vi "read_channels_specify_range.vi"(5 "postDAQ  wait ms":u32=12, 7 "preDAQ  wait ms":u32=25, 8 "error in":T1, 11 "K6517 GPIB Address":string) -> (0 "error out":T1, 2 "data":dbl[](array[numeric]), 3 "K6517 GPIB Address out":string)   [LabVIEW 2024]
uses:
  <instrlib>/Keithley 6517/Keithley 6517.lvlib
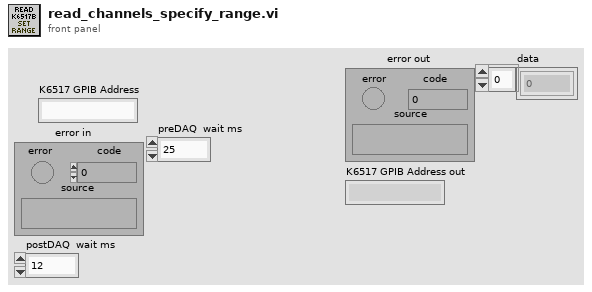
[diagram p1: front panel]
types:
  T1 = cluster{"error":bool, "code":i32, "source":string}
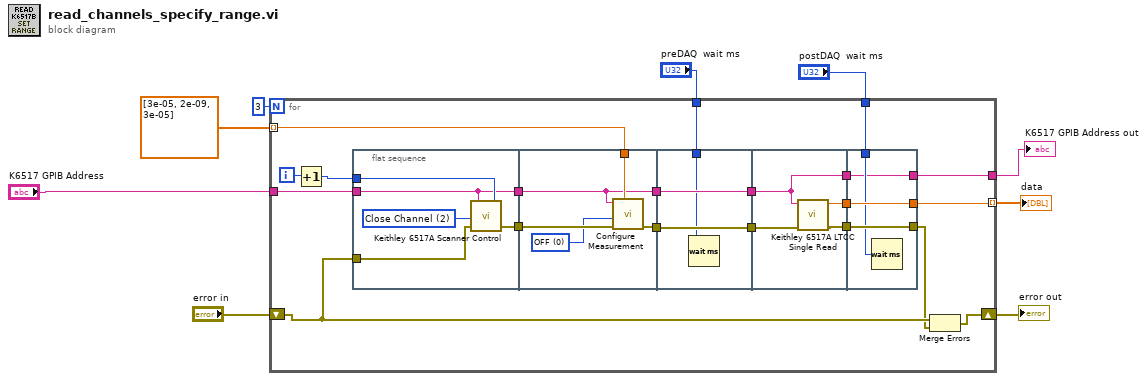
[diagram p0: block diagram]
diagram:
  n1 = for {
    N: 3 -> [_]
    tunnel: "K6517 GPIB Address" -> [w26]
    shift-right: [w29] -> w2
    shift-left: "error in" -> [w25]
    tunnel: dbl[] [3e-05, 2e-09, 3e-05] -> [w24] mode=indexing
    tunnel: [w14] -> w3 mode=indexing
    tunnel: "preDAQ  wait ms" -> [w13]
    tunnel: "postDAQ  wait ms" -> [w12]
    tunnel: [w11] -> w1
    i -> [w28]
    n2 = Increment(x=w28) -> (x+1=w27:i32)
    n3 = flat-sequence {
      tunnel: w27 -> [w33]
      tunnel: w26 -> [w31]
      tunnel: w25 -> [w32]
      tunnel: [w31] -> w23
      tunnel: [w30] -> w22
      tunnel: w24 -> [w37]
      tunnel: [w36] -> w20
      tunnel: [w35] -> w18
      tunnel: w22 -> [w39]
      tunnel: w23 -> [w35]
      tunnel: w20 -> [w42]
      tunnel: [w42] -> w19
      tunnel: w18 -> [w41]
      tunnel: [w41] -> w17
      tunnel: w13 -> [w40]
      tunnel: w19 -> [w46]
      tunnel: w17 -> [w43]
      tunnel: [w45] -> w21
      tunnel: [w44] -> w15
      tunnel: [w43] -> w10
      tunnel: [w50] -> w16
      tunnel: w21 -> [w50]
      tunnel: [w49] -> w14
      tunnel: w15 -> [w49]
      tunnel: w12 -> [w48]
      tunnel: [w47] -> w11
      tunnel: w10 -> [w47]
      frame #0 {
        w34 = u16 2 items=["Open All", "Open Channel", "Close Channel", "Scan List"] ("Scanner Control")
        n4 = call "Keithley 6517A Scanner Control.vi"("Open / Close Internal Scanner Channel"=w33, "error in"=w32, "Scanner Control"=w34, "GPIB address"=w31) -> ("error out"=w30:T1)  [unwired: 1 in]
      }
      frame #1 {
        w38 = 0 items=["OFF", "ON", "ONCE"] ("Auto Range (1: ON)")
        n5 = call <instrlib>:"Configure Measurement.vi"("Auto Range Value (2.0000000E+2)"=w37, "error in (no error)"=w39, "Auto Range (1: ON)"=w38, "VISA resource name"=w35) -> ("error out"=w36:errorcluster)  [unwired: 6 in, 1 out]
      }
      frame #2 {
        n6 = Wait (ms)(milliseconds to wait=w40) -> ()  [unwired: 1 out]
      }
      frame #3 {
        n7 = call "Keithley 6517A LTCC Single Read.vi"("error in"=w46, "GPIB address"=w43) -> ("error out"=w45:T1, "measurement"=w44:dbl)  [unwired: 2 in, 6 out]
      }
      frame #4 {
        n8 = Wait (ms)(milliseconds to wait=w48) -> ()  [unwired: 1 out]
      }
    }
    n9 = Merge Errors(w25, w16) -> (w29:errorcluster)
  }
  "error out" <- w2
  "data" <- w3
  "K6517 GPIB Address out" <- w1
